vi "AlliGator Fit Method Benchmark.vi"() -> ()   [LabVIEW 2021, in "AlliGator Fit Method Benchmark.lvlib"]
doc: "Fit Method Benchmark GUI."
uses:
  AlliGator Fit Method Benchmark.lvlib
  AlliGator Fit Simulation Parameters.ctl
  AlliGator Decay Simulation Parameters.ctl
  Arrays/Array Statistics.ctl
  Fits/Decay Convolution/Decay Model.ctl
  Fits/Residual Type.ctl
  Fits/IRF(X)PSED/Fit Weights Type.ctl
  Fits/Non-linear Fitting Method v2.ctl
  Fits/Fit Calculation Method.ctl
  Fits/Non-linear Fitting Algorithm.ctl
  AlliGator Decay Fit Parameter Constraints 2.ctl
  Fits/IRF(X)PSED/Decay Fit Parameters In List.ctl
  Fits/IRF(X)PSED/MLE Baseline Offset Type.ctl
  Fits/IRF(X)PSED/IRF(X)PSED Fit Results.ctl
  AlliGator Decay Fit Options & Parameters v2.ctl
  Fits/IRF(X)PSED/Decay Fit Options v2.ctl
  Graphs/XY Graph/XY Graph Event.ctl
  <vilib>/Utility/miscctls.llb/LVPoint32TypeDef.ctl
  1e2fc33e-f2e1-4865-bd35-b782600da79c.vi
  ffbda573-fdee-4728-9e4a-091745fb94a5.vi
  20485d49-49ee-422f-9a66-761cdf75a503.vi
  AlliGator Abort.vi
  Graphs/XY Graph/XY Graph Add Single Plot with Name.vi
  GUI/GUI.lvlib
  Notebook/Notebook.lvlib
  Error/Error.lvlib
  AlliGator Globals, Variables & Constants.lvlib
  Graphs/XY Graph/XY Graph Add-Ons.lvlib
  Fits/Fits.lvlib
  AlliGator Decay Fit.lvlib
  AlliGator Decay Fit Parameter Map.lvlib
  Utilities/Utilities.lvlib
  <vilib>/vision/NI_Vision_Development_Module.lvlib
  Arrays/Arrays.lvlib
panel:
  in  "Tab Control":T1(tab)
  in  "Export Results":bool
  in  "Histogram Lower Percentile":dbl
  in  "Histogram Upper Percentile":dbl=100.0
  out "Histograms":cluster{"Axis":dbl[], "Histogram":dbl[]}[](graph)
  in  "Run Simulation":bool
  in  "Fit Simulation Parameters":T2={"# Counts"=100, "# Simulations (N)"=100, "Decay Bin Size"=1.0000000000000002e-10, "# Bins"=200}
  in  "Decay Simulation Parameters":T3={"tau 1"=1e-09, "tau 2"=0.0, "a1"=1.0, "Baseline"=0.0}
  out "tau 1":T4 {"Min" format="%#_4g"; "Max" format="%#_4g"; "Mean" format="%#_4g"; "Standard Deviation" format="%#_4g"}
  out "tau 2":T4 {"Min" format="%#_4g"; "Max" format="%#_4g"; "Mean" format="%#_4g"; "Standard Deviation" format="%#_4g"}
  out "a1":T4 {"Min" format="%#_4g"; "Max" format="%#_4g"; "Mean" format="%#_4g"; "Standard Deviation" format="%#_4g"}
  out "Message":string caption="Output (see Notebook)"
  in  "Histogram Bin Size (a1)":dbl=0.1
  in  "Histogram Bin Size (Lifetime)":dbl[unit]=1.0000000000000002e-10
  out "# Photons":dbl[](array[numeric])
  in  "Select Decay, Fit & Residuals Index":i32=1 min=1
  out "Decay Graph":cluster{"Axis":dbl[], "Histogram":dbl[]}[](graph)
  in  "Show Decays, Fits & Residuals":bool
  out "Experimental IRF Loaded":bool
  in  "Use Experimental IRF":bool
  in  "# Logical Processors Used":i32=4 caption="Used" min=1 max=16
  out "# Logical Processors":i32
  in  "MLE Baseline Offset Type":T5
  in  "MLE Baseline Offset":dbl
  in  "Fit Parameter Constraints":T6[](array[typedef]) {"Max Value" format="%#.3g"; "Min Value" format="%#.3g"}
  in  "Decay Fit Options":T14={"Show Fit Residuals"=TRUE, "Fit Model"=enum."1-Exponential", "Residual Type"=enum."Standard", "Max Decay Percentile"=100.0, "Min Decay Percentile"=0.0, "Show Full Decay"=TRUE, "Weights"=enum."1/Variance", "Fitting Method"=enum."Least Square", "Compute Parameter Uncertainties"=TRUE, "Periodic Boundaries"=TRUE, "Model Calculation"=enum."Simulation", "Period"=1.2500000000000001e-08, "Termination Criteria"={"Max Iterations"=1000, "Max Function Calls"=10000, "Max Time"=100.0, "Function Tolerance"=1e-06, "Parameter Tolerance"=1e-06, "Gradient Tolerance"=1e-06, "Min Lambda"=1e-06, "Max Lambda"=1000000.0, "Initial Tick Count"=0}, "Offset Resolution"=5.000000000000001e-11, "Use Local IRF"=FALSE, "Fitting Algorithm"=enum."Levenberg-Marquardt"} {"Offset Resolution" min=0.0; "Period" min=0.0; "Min Decay Percentile" min=0.0 max=1.0; "Max Decay Percentile" min=0.0 max=100.0}
  in  "Animated Busy Icon":bool=TRUE
  in  "Abort":bool
  out "Progress Bar":dbl(slide) scale=0.0..100.0
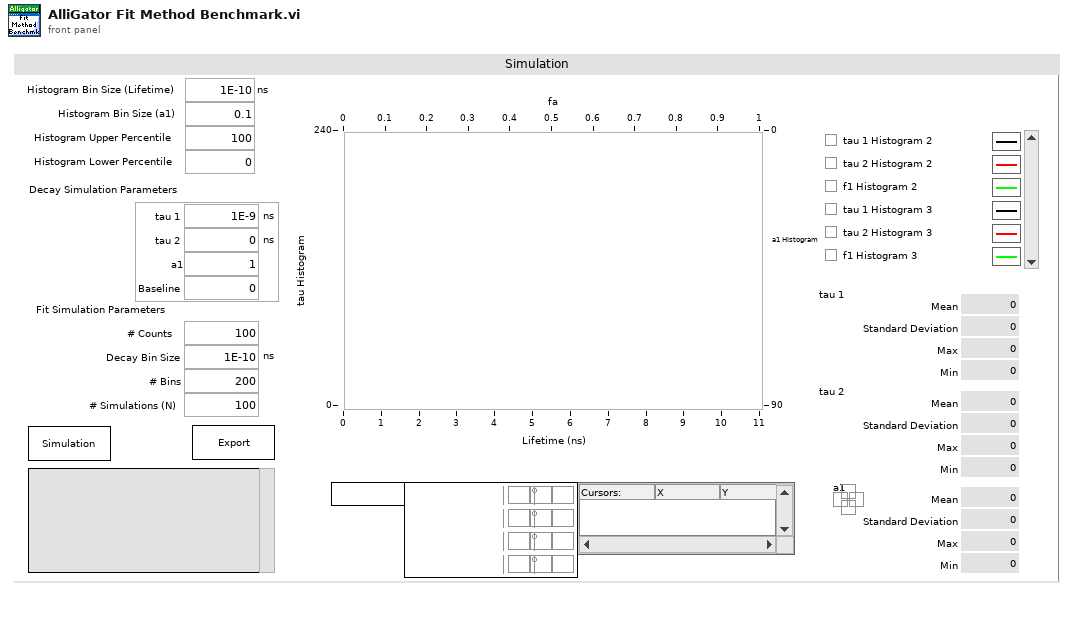
[diagram p1: front panel]
types:
  T1 = enum32{"Simulation", "Decay, Fit & Residuals Plots", "Settings"}
  T2 = typedef "AlliGator Fit Method Benchmark.lvlib/AlliGator Fit Simulation Parameters.ctl" = cluster{"# Counts":i32, "# Simulations (N)":i32, "Decay Bin Size":dbl[unit], "# Bins":i32}
  T3 = typedef "AlliGator Fit Method Benchmark.lvlib/AlliGator Decay Simulation Parameters.ctl" = cluster{"tau 1":dbl[unit], "tau 2":dbl[unit], "a1":dbl, "Baseline":dbl}
  T4 = typedef "Arrays.lvlib/Array Statistics.ctl" = cluster{"Mean":dbl, "Standard Deviation":dbl, "Max":dbl, "Min":dbl}
  T5 = typedef "Fits.lvlib/MLE Baseline Offset Type.ctl" = enum32{"Absolute", "Percentage"}
  T6 = typedef "AlliGator Decay Analysis.lvlib/AlliGator Decay Fit.lvlib/AlliGator Decay Fit Parameter Constraints 2.ctl" = cluster{"Fit Parameter":T7, "Min Value":dbl, "Max Value":dbl, "Global":bool, "Used":bool}
  T7 = typedef "Fits.lvlib/Decay Fit Parameters In List.ctl" = enum16{"Offset", "Baseline", "A_1", "tau_1", "A_2", "tau_2"}
  T8 = typedef "Fits.lvlib/Decay Model.ctl" = enum16{"1-Exponential", "2-Exponentials"}
  T9 = typedef "Fits.lvlib/Residual Type.ctl" = enum16{"Standard", "Normalized", "Reduced"}
  T10 = typedef "Fits.lvlib/Fit Weights Type.ctl" = enum16{"Unweighted", "1/Variance", "Best of All"}
  T11 = typedef "Fits.lvlib/Non-linear Fitting Method v2.ctl" = enum16{"Least Square", "Least Absolute Residual", "Bisquare", "MLE", "-", "Best of All"}
  T12 = typedef "Fits.lvlib/Fit Calculation Method.ctl" = enum16{"Simulation", "Convolution", "Integration"}
  T13 = typedef "Fits.lvlib/Non-linear Fitting Algorithm.ctl" = enum16{"Levenberg-Marquardt", "Trust-Region Dogleg"}
  T14 = cluster{"Show Fit Residuals":bool, "Fit Model":T8, "Residual Type":T9, "Max Decay Percentile":dbl, "Min Decay Percentile":dbl, "Show Full Decay":bool, "Weights":T10, "Fitting Method":T11, "Compute Parameter Uncertainties":bool, "Periodic Boundaries":bool, "Model Calculation":T12, "Period":dbl[unit], "Termination Criteria":cluster{"Max Iterations":i32, "Max Function Calls":i32, "Max Time":dbl[unit], "Function Tolerance":dbl, "Parameter Tolerance":dbl, "Gradient Tolerance":dbl, "Min Lambda":dbl, "Max Lambda":dbl, "Initial Tick Count":u32}, "Offset Resolution":dbl[unit], "Use Local IRF":bool, "Fitting Algorithm":T13}
  T15 = typedef "XY Graph Add-Ons.lvlib/XY Graph Refnum.ctl" = refnum<vi>
  T16 = typedef "AlliGator Progress Bar Q Element.ctl" = cluster{"Action":string, "Value":dbl}
  T17 = typedef "Fits.lvlib/IRF(X)PSED Fit Results.ctl" = cluster{"Best Fit Parameters (All)":dbl[], "Delta Best Fit Parameters (All)":dbl[], "R^2":dbl, "Reduced Chi^2":dbl}
  T18 = typedef "AlliGator Decay Fit Parameter Map.lvlib/AlliGator Decay Fit Options & Parameters v2.ctl" = cluster{"SYNC Period":dbl[unit], "Fit Options":T19, "Fit Parameter Constraints":T6[], "MLE Baseline Offset":dbl, "MLE Baseline Offset Type":T5}
  T19 = typedef "Fits.lvlib/Decay Fit Options v2.ctl" = cluster{"Show Fit Residuals":bool, "Fit Model":T8, "Residual Type":T9, "Max Decay Percentile":dbl, "Min Decay Percentile":dbl, "Show Full Decay":bool, "Weights":T10, "Fitting Method":T11, "Compute Parameter Uncertainties":bool, "Periodic Boundaries":bool, "Model Calculation":T12, "Period":dbl[unit], "Termination Criteria":cluster{"Max Iterations":i32, "Max Function Calls":i32, "Max Time":dbl[unit], "Function Tolerance":dbl, "Parameter Tolerance":dbl, "Gradient Tolerance":dbl, "Min Lambda":dbl, "Max Lambda":dbl, "Initial Tick Count":u32}, "Offset Resolution":dbl[unit], "Use Local IRF":bool, "Fitting Algorithm":T13}
  T20 = typedef "XY Graph Add-Ons.lvlib/XY Graph Event.ctl" = cluster{"Item Tag":string, "XY Graph Refnum":refnum<vi>, "Coords":T21, "Item Path":string}
  T21 = typedef "LVPoint32TypeDef.ctl" = cluster{"Horizontal":i32, "Vertical":i32}
  T22 = typedef "XY Graph Add-Ons.lvlib/XY Plot Data.ctl" = cluster{"X Array":dbl[], "Y Array":dbl[]}
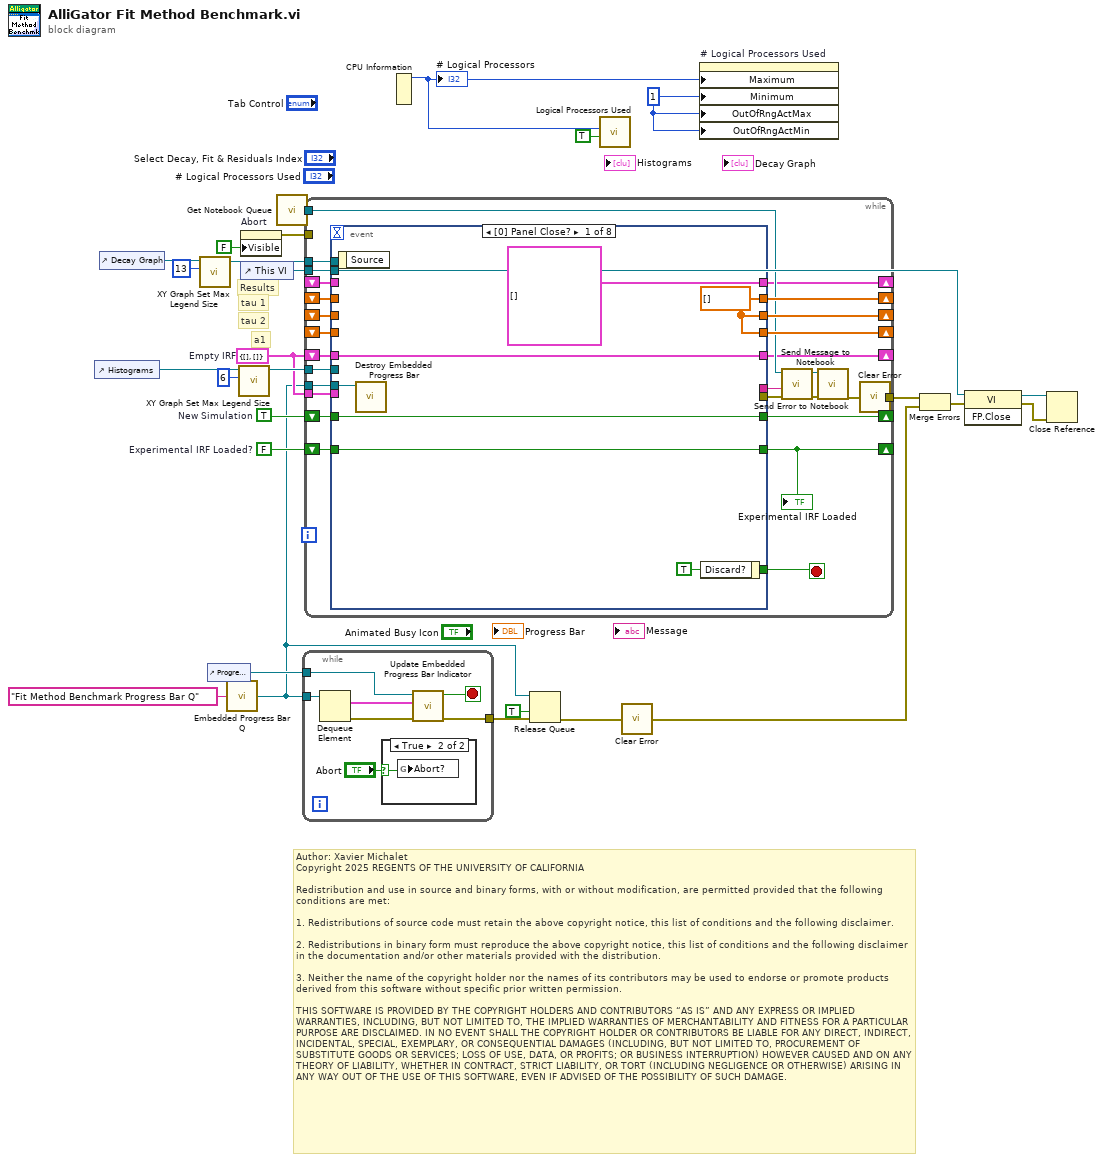
[diagram p0: block diagram]
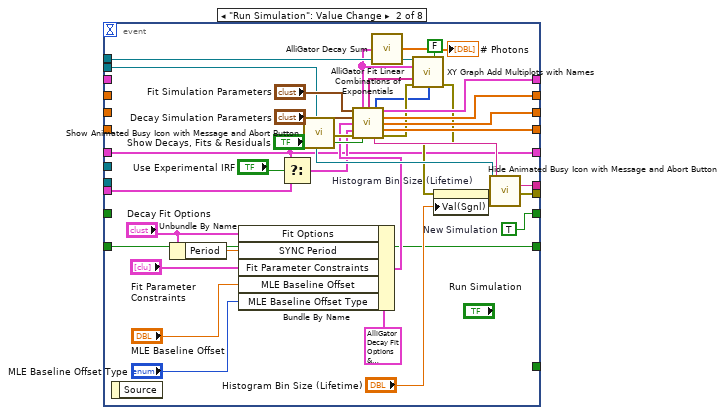
[diagram p3: hidden frame]
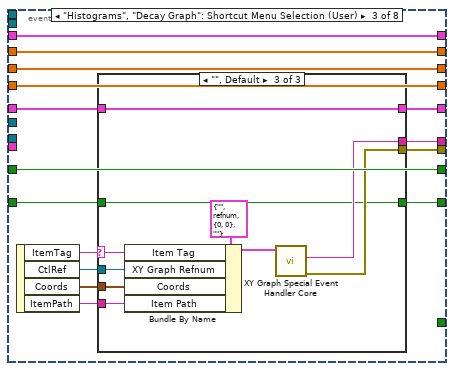
[diagram p4: hidden frame]
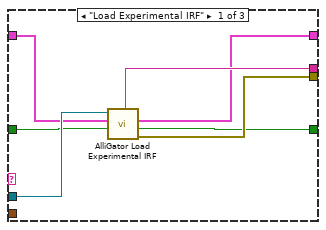
[diagram p5: hidden frame]
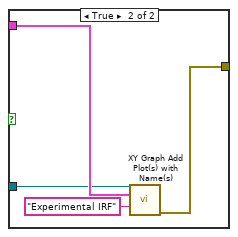
[diagram p7: hidden frame]
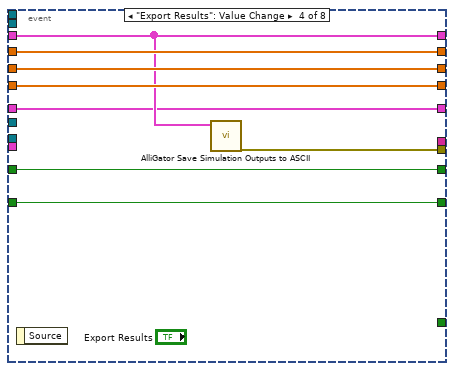
[diagram p8: hidden frame]
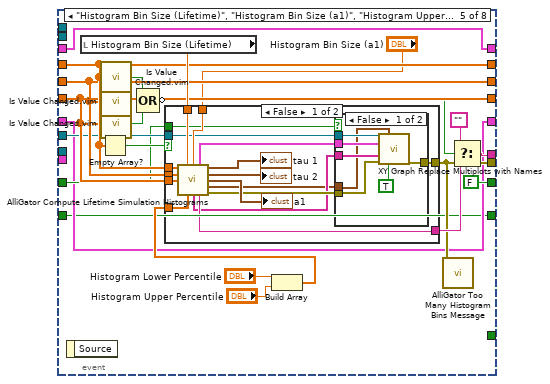
[diagram p9: hidden frame]
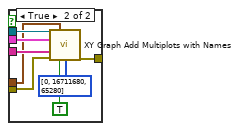
[diagram p10: hidden frame]
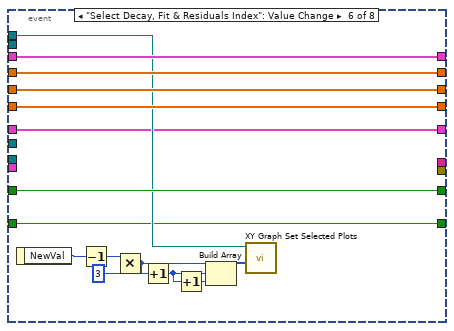
[diagram p12: hidden frame]
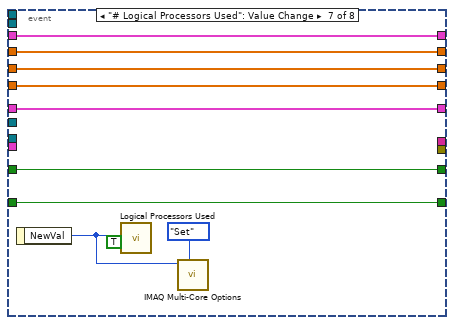
[diagram p13: hidden frame]
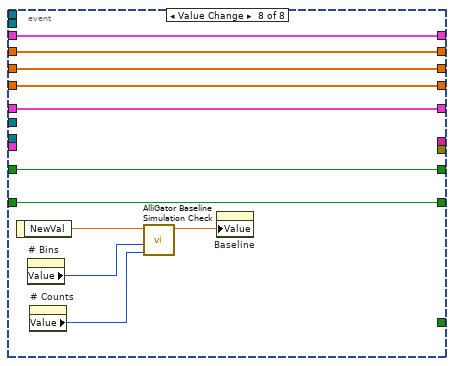
[diagram p14: hidden frame]
diagram:
  w3 = FALSE  # Experimental IRF Loaded?
  w4 = cluster{"t Array":dbl[], "IRF Array":dbl[]} {"t Array"=[], "IRF Array"=[]}  # Empty IRF
  w5 = u8 1 ("Data Entry Limits:Minimum")
  w8 = TRUE  # New Simulation
  # "Author: Xavier Michalet\nCopyright 2025 REGENTS OF THE UNIVERSITY OF CALIFORNIA\n\nRedistribution and use in source and binary forms, with or without modification, are permitted provided that the following conditions are met:\n\n1. Redistributions of source code must retain the above copyright notice, this list of conditions and the following disclaimer.\n\n2. Redistributions in binary form must reproduce the above copyright notice, this list of conditions and the following disclaimer in the documentation and/or other materials provided with the distribution.\n\n3. Neither the name of the copyright holder nor the names of its contributors may be used to endorse or promote products derived from this software without specific prior written permission.\n\nTHIS SOFTWARE IS PROVIDED BY THE COPYRIGHT HOLDERS AND CONTRIBUTORS “AS IS” AND ANY EXPRESS OR IMPLIED WARRANTIES, INCLUDING, BUT NOT LIMITED TO, THE IMPLIED WARRANTIES OF MERCHANTABILITY AND FITNESS FOR A PARTICULAR PURPOSE ARE DISCLAIMED. IN NO EVENT SHALL THE COPYRIGHT HOLDER OR CONTRIBUTORS BE LIABLE FOR ANY DIRECT, INDIRECT, INCIDENTAL, SPECIAL, EXEMPLARY, OR CONSEQUENTIAL DAMAGES (INCLUDING, BUT NOT LIMITED TO, PROCUREMENT OF SUBSTITUTE GOODS OR SERVICES; LOSS OF USE, DATA, OR PROFITS; OR BUSINESS INTERRUPTION) HOWEVER CAUSED AND ON ANY THEORY OF LIABILITY, WHETHER IN CONTRACT, STRICT LIABILITY, OR TORT (INCLUDING NEGLIGENCE OR OTHERWISE) ARISING IN ANY WAY OUT OF THE USE OF THIS SOFTWARE, EVEN IF ADVISED OF THE POSSIBILITY OF SUCH DAMAGE."
  # "Results"
  # "a1"
  # "tau 2"
  # "tau 1"
  n1 = control-ref of="Histograms"() -> (w14:refnum<vi>)
  n2 = control-ref of="Decay Graph"() -> (w11:refnum<vi>)
  n3 = call "XY Graph Set Max Legend Size.vi"("Max Legend Size"=13, "XY Graph Refnum"=w11) -> ("XY Graph Refnum (dup)"=w10:T15)  [unwired: 8 in, 1 out]
  n4 = control-ref of="Progress Bar"() -> (w26:refnum<vi>)
  n5 = call "Embedded Progress Bar Q.vi"("Progress Bar Queue Name"="Fit Method Benchmark Progress Bar Q") -> ("Progress Bar Queue"=w1:refnum<queue>)  [unwired: 6 in]
  n6 = call "XY Graph Set Max Legend Size.vi"("Max Legend Size"=6, "XY Graph Refnum"=w14) -> ("XY Graph Refnum (dup)"=w12:T15)  [unwired: 8 in, 1 out]
  n7 = property on="Abort" class="Bool"("Visible"=FALSE) -> (error out=w16:errorcluster)  [unwired: 2 in, 1 out]
  n8 = control-ref of="This VI"() -> (w15:refnum<vi>)
  n9 = call "Get Notebook Queue.vi"() -> ("Notebook Queue"=w23:refnum<queue>)  [unwired: 9 in]
  n10 = while {
    tunnel: w1 -> [w34]
    tunnel: w26 -> [w32]
    tunnel: [w29] -> w25
    stop <- w30 stop-if-true
    n11 = Dequeue Element(queue=w34) -> (element=w33:T16, error out=w31:errorcluster)  [unwired: 2 in, 2 out]
    n12 = case shown="True" "Abort" {
      selector: "Abort" -> [_ w35]
      frame False {
      }
      frame True {
        n13 = global write "AlliGator Abort.vi" "Abort?"(w35) -> ()
      }
    }
    n14 = call "Update Embedded Progress Bar Indicator.vi"("Error In"=w31, "Progress Bar Event"=w33, "Progress Bar Refnum"=w32) -> ("Error Out"=w29:errorcluster, "Quit?"=w30:bool)  [unwired: 7 in]
  }
  n15 = while {
    shift-right: [w61] -> _
    shift-left: _ -> [w58]
    shift-right: [w60] -> _
    shift-left: _ -> [w57]
    shift-right: [w59] -> _
    shift-left: _ -> [w56]
    tunnel: w1 -> [w55]
    tunnel: w23 -> [w54]
    tunnel: [w48] -> w22
    tunnel: w16 -> [_]
    tunnel: w15 -> [w47]
    tunnel: w12 -> [w46]
    shift-right: [w45] -> _
    shift-left: _ -> [w44]
    tunnel: w10 -> [w43]
    shift-right: [w41] -> _
    shift-left: w8 -> [w42]
    shift-right: [w39] -> _
    shift-left: w4 -> [w40]
    tunnel: w4 -> [w38]
    shift-right: [w36] -> _
    shift-left: w3 -> [w37]
    stop <- w62 stop-if-true
    n16 = event shown="[0] Panel Close?" {
      selector: _ -> [_ _ _ _ _ _ _ _]
      dyn-events: _ -> [_ _ _ _ _ _ _ _]
      timeout: _ -> [_ _ _ _ _ _ _ _]
      tunnel: [w69 _ _ _ _ _ _ _] -> w62
      tunnel: [w66 w101 w118 w151 w172 w221 w231 w242] -> w61
      tunnel: [w66 w100 w117 w150 w171 w220 w230 w241] -> w60
      tunnel: [w66 w99 w116 w149 w170 w219 w229 w240] -> w59
      tunnel: w58 -> [_ _ w118 w151 w172 w221 w231 w242]
      tunnel: w57 -> [_ _ w117 w150 w171 w220 w230 w241]
      tunnel: w56 -> [_ _ w116 w149 w170 w219 w229 w240]
      tunnel: w55 -> [w68 _ _ _ _ _ _ _]
      tunnel: [_ w94 w111 _ w164 _ _ _] -> w53
      tunnel: [_ w95 w110 w146 w154 _ _ _] -> w49
      tunnel: w47 -> [_ w82 _ _ _ _ _ _]
      tunnel: w46 -> [_ _ _ _ w159 _ _ _]
      tunnel: [T17[] [] ("Fit Results") w89 w109 w147 w158 w218 w228 w239] -> w45
      tunnel: w44 -> [_ _ w109 w147 w158 w218 w228 w239]
      tunnel: w43 -> [_ w86 _ _ _ w216 _ _]
      tunnel: w42 -> [w65 _ w108 w148 w156 w217 w227 w238]
      tunnel: [w65 w78 w108 w148 FALSE ("New Simulation") w217 w227 w238] -> w41
      tunnel: w40 -> [w64 w74 w107 w145 w153 w208 w223 w233]
      tunnel: [w64 w74 w106 w145 w153 w208 w223 w233] -> w39
      tunnel: w38 -> [_ w73 _ _ _ _ _ _]
      tunnel: w37 -> [w63 w72 w105 w144 w152 w207 w222 w232]
      tunnel: [w63 w72 w104 w144 w152 w207 w222 w232] -> w36
      event Panel Close? {
        w66 = dbl[] [] ("tau 1")
        w69 = TRUE ("Discard?")
        n17 = event-data() -> ()  [unwired: 1 in, 1 out]
        n18 = call "Destroy Embedded Progress Bar.vi"("Progress Bar Queue in"=w68) -> ()  [unwired: 10 in, 1 out]
        n19 = event-data("Discard?"=w69) -> ()  [unwired: 1 in, 1 out]
      }
      event "Run Simulation": Value Change {
        w78 = TRUE  # New Simulation
        n20 = event-data() -> ()  [unwired: 1 in, 1 out]
        n21 = Unbundle By Name("Decay Fit Options") -> ("Period"=w93:dbl[unit])
        n22 = Bundle By Name(cluster=T18 {"SYNC Period"=0.0, "Fit Options"={"Show Fit Residuals"=FALSE, "Fit Model"=enum."1-Exponential", "Residual Type"=enum."Standard", "Max Decay Percentile"=0.0, "Min Decay Percentile"=0.0, "Show Full Decay"=FALSE, "Weights"=enum."Unweighted", "Fitting Method"=enum."Least Square", "Compute Parameter Uncertainties"=FALSE, "Periodic Boundaries"=FALSE, "Model Calculation"=enum."Simulation", "Period"=0.0, "Termination Criteria"={"Max Iterations"=0, "Max Function Calls"=0, "Max Time"=0.0, "Function Tolerance"=0.0, "Parameter Tolerance"=0.0, "Gradient Tolerance"=0.0, "Min Lambda"=0.0, "Max Lambda"=0.0, "Initial Tick Count"=0}, "Offset Resolution"=0.0, "Use Local IRF"=FALSE, "Fitting Algorithm"=enum."Levenberg-Marquardt"}, "Fit Parameter Constraints"=[], "MLE Baseline Offset"=0.0, "MLE Baseline Offset Type"=enum."Absolute"} ("Decay Fit Options & Parameters"), "Fit Options"="Decay Fit Options", "SYNC Period"=w93, "Fit Parameter Constraints"="Fit Parameter Constraints", "MLE Baseline Offset"="MLE Baseline Offset", "MLE Baseline Offset Type"="MLE Baseline Offset Type") -> (w81:T18)
        n23 = Select(t=w74, s="Use Experimental IRF", f=w73) -> (s? t:f=w75:T22)
        n24 = call "Show Animated Busy Icon with Message and Abort Button.vi"("Target VI reference"=w82) -> ("Error Out"=w97:errorcluster)  [unwired: 18 in]
        n25 = call "AlliGator Fit Linear Combinations of Exponentials.vi"("Fit Simulation Parameters"="Fit Simulation Parameters", "Decay Simulation Parameters"="Decay Simulation Parameters", "Decay Fit Options & Parameters"=w81, "Reference Decay"=w75, "Error In"=w97, "Show Decays, Fits & Residuals"="Show Decays, Fits & Residuals") -> ("Output Plots"=w71:cluster{"t Array":dbl[], "I Array":dbl[]}[], "Output Plot Names"=w85:string[], "Plot Colors"=w84:u32[], "Fit Results"=w89:T17[], "tau 1"=w101:dbl[], "tau 2"=w100:dbl[], "a 1"=w99:dbl[], "Message"=w94:string, "Error Out"=w87:errorcluster)  [unwired: 1 in]
        n26 = call "AlliGator Decay Sum.vi"("Output Plots"=w71) -> ("# Photons"=→"# Photons":dbl[])
        n27 = call "XY Graph Add Multiplots with Names.vi"("XYGraph in"=w86, "Keep Existing Plots (T)"=FALSE, "Array of Plots"=w71, "Array of Plot Names (\"Plot\")"=w85, "error in (no error)"=w87, "Plot Colors (Default)"=w84) -> ("error out"=w77:errorcluster)  [unwired: 5 in, 4 out]
        n28 = property on="Histogram Bin Size (Lifetime)" class="DigNum (strict)"(error in=w77, "Val(Sgnl)"="Histogram Bin Size (Lifetime)") -> (error out=w96:errorcluster)  [unwired: 1 in, 1 out]
        n29 = call "Hide Animated Busy Icon with Message and Abort Button.vi"("Message"=w94, "Target VI reference"=w82, "Error In"=w96) -> ("Error Out"=w95:errorcluster)  [unwired: 16 in]
      }
      event "Histograms", "Decay Graph": Shortcut Menu Selection (User) {
        n30 = event-data() -> ("ItemTag"=w115:string, "CtlRef"=w114:refnum<vi>, "Coords"=w113:T21, "ItemPath"=w112:string)  [unwired: 1 in]
        n31 = case shown="\"\", Default" w115 {
          selector: w115 -> [_ _ w142]
          tunnel: w114 -> [w125 w127 w141]
          tunnel: w113 -> [_ _ w140]
          tunnel: w112 -> [_ _ w139]
          tunnel: [w123 _ w137] -> w111
          tunnel: [w124 w126 w136] -> w110
          tunnel: w107 -> [w120 w128 w135]
          tunnel: [w119 w128 w135] -> w106
          tunnel: w105 -> [w121 w129 w134]
          tunnel: [w122 w129 w134] -> w104
          frame "Load Experimental IRF" {
            n32 = call "AlliGator Load Experimental IRF.vi"("Experimental IRF Loaded?"=w121, "Plot Data in"=w120, "XYGraph in"=w125) -> ("error out"=w124:errorcluster, "Experimental IRF Loaded?"=w122:bool, "Plot Data out"=w119:T22, "Message"=w123:string)  [unwired: 5 in]
          }
          frame "Show Experimental IRF" {
            n33 = case shown="False" w129 {
              tunnel: w128 -> [_ w133]
              tunnel: w127 -> [_ w132]
              tunnel: [_ w130] -> w126
              frame False {
              }
              frame True {
                n34 = call-poly "XY Graph Add Plot(s) with Name(s).vi"("XYGraph Ref in"=w132, "Plot"=w133, "Plot Name (\"Plot\")"="Experimental IRF" ("Plot Name (\"Plot\")")) -> ("error out"=w130:errorcluster)  [unwired: 9 in, 3 out]
              }
            }
          }
          frame "", Default {
            n35 = Bundle By Name(cluster=T20 {"Item Tag"="", "XY Graph Refnum"=refnum, "Coords"={"Horizontal"=0, "Vertical"=0}, "Item Path"=""} ("XY Graph Event"), "Item Tag"=w142, "XY Graph Refnum"=w141, "Coords"=w140, "Item Path"=w139) -> (w138:T20)
            n36 = call "XY Graph Special Event Handler Core.vi"("XY Graph Event"=w138) -> ("error out"=w136:errorcluster, "Message"=w137:string)  [unwired: 6 in, 3 out]
          }
        }
      }
      event "Export Results": Value Change {
        n37 = event-data() -> ()  [unwired: 1 in, 1 out]
        n38 = call "AlliGator Save Simulation Outputs to ASCII.vi"("Fit Results"=w147) -> ("Error Out"=w146:errorcluster)  [unwired: 10 in]
      }
      event "Histogram Bin Size (Lifetime)", "Histogram Bin Size (a1)", "Histogram Upper Percentile", "Histogram Lower Percentile": Value Change {
        n39 = event-data() -> ()  [unwired: 1 in, 1 out]
        n40 = local read "Histogram Bin Size (Lifetime)"() -> (w174:dbl[unit])
        n41 = Empty Array?(array=w172) -> (empty?=w173:bool)
        n42 = call "Is Value Changed.vim"("value"=w172) -> ("changed or first call?"=w169:bool)
        n43 = call "Is Value Changed.vim"("value"=w171) -> ("changed or first call?"=w168:bool)
        n44 = call "Is Value Changed.vim"("value"=w170) -> ("changed or first call?"=w167:bool)
        n45 = Compound Arithmetic op=OR(w169, w168, w167) -> (invert w166:bool)
        n46 = Build Array("Histogram Lower Percentile", "Histogram Upper Percentile") -> (w160:dbl[])
        n47 = case shown="False" w173 {
          tunnel: w174 -> [w191 _]
          tunnel: w171 -> [w190 _]
          tunnel: w170 -> [w189 _]
          tunnel: w172 -> [w188 _]
          tunnel: [w184 _] -> w165
          tunnel: [w178 _] -> w154
          tunnel: "Histogram Bin Size (a1)" -> [w183 _]
          tunnel: w160 -> [w182 _]
          tunnel: w159 -> [w181 _]
          tunnel: w156 -> [w176 _]
          frame False {
            n48 = call "AlliGator Compute Lifetime Simulation Histograms.vi"("tau 1"=w188, "Histogram Bin Size (tau)"=w191, "Histogram Bin Size (f1)"=w183, "tau 2"=w190, "a1"=w189, "Percentiles to Keep (1, 99)"=w182) -> ("Histograms"=w180:cluster{"Axis":dbl[], "Histogram":dbl[]}[], "Array Statistic (tau 1)"=→"tau 1":T4, "Array Statistics (tau 2)"=→"tau 2":T4, "Array Statistics (a1)"=→"a1":T4, "Array of Scales"=w175:cluster{"X Scale":u32, "Y Scale":u32}[], "Plot Names"=w177:string[], "Message"=w184:string, "Error Out"=w179:errorcluster)  [unwired: 2 in]
            n49 = case shown="False" w176 {
              tunnel: w181 -> [w198 w206]
              tunnel: w180 -> [w197 w205]
              tunnel: w179 -> [w195 w204]
              tunnel: [w194 w203] -> w178
              tunnel: w177 -> [w196 w201]
              tunnel: w175 -> [w192 w200]
              frame False {
                n50 = call "XY Graph Replace Multiplots with Names.vi"("XYGraph in"=w198, "Array of Scales (Default)"=w192, "Array of Plots"=w197, "Array of Plot Names (\"Plot\")"=w196, "error in (no error)"=w195, "Make Visible (T)"=TRUE) -> ("error out"=w194:errorcluster)  [unwired: 5 in, 4 out]
              }
              frame True {
                n51 = call "XY Graph Add Multiplots with Names.vi"("XYGraph in"=w206, "Array of Scales (Default)"=w200, "Array of Plots"=w205, "Array of Plot Names (\"Plot\")"=w201, "error in (no error)"=w204, "Make Visible (T)"=TRUE, "Plot Colors (Default)"=u32[] [0, 16711680, 65280]) -> ("error out"=w203:errorcluster)  [unwired: 4 in, 4 out]
              }
            }
          }
          frame True {
          }
        }
        n52 = call "AlliGator Too Many Histogram Bins Message.vi"("error in (no error)"=w154) -> ()
        n53 = Select(t="", s=w166, f=w165) -> (s? t:f=w164:string)
      }
      event "Select Decay, Fit & Residuals Index": Value Change {
        n54 = event-data() -> ("NewVal"=w215:i32)  [unwired: 1 in]
        n55 = Decrement(x=w215) -> (x-1=w214:i32)
        n56 = Multiply(x=w214, y=3) -> (x*y=w211:i32)
        n57 = Increment(x=w211) -> (x+1=w210:i32)
        n58 = Increment(x=w210) -> (x+1=w209:i32)
        n59 = Build Array(w211, w210, w209) -> (w212:i32[])
        n60 = call "XY Graph Set Selected Plots.vi"("Selected Plots"=w212, "XY Graph Refnum"=w216) -> ()  [unwired: 6 in, 4 out]
      }
      event "# Logical Processors Used": Value Change {
        n61 = event-data() -> ("NewVal"=w224:i32)  [unwired: 1 in]
        n62 = call "Logical Processors Used.vi"("Set/Get (F)"=TRUE, "# Logical Processor Used"=w224) -> ()  [unwired: 4 in, 1 out]
        n63 = call "IMAQ Multi-Core Options"("Get/Set Number of Cores (Get)"=enum32{"Get", "Set", "Set Max Available"}."Set", "Specified Number of Cores"=w224) -> ()  [unwired: 8 in, 2 out]
      }
      event Value Change {
        n64 = event-data() -> ("NewVal"=w237:dbl)  [unwired: 1 in]
        n65 = property on="# Bins" class="DigNum (strict)"() -> ("Value"=w236:i32)  [unwired: 2 in, 2 out]
        n66 = property on="# Counts" class="DigNum (strict)"() -> ("Value"=w235:i32)  [unwired: 2 in, 2 out]
        n67 = call "AlliGator Baseline Simulation Check.vi"("# Counts"=w235, "# Bins"=w236, "New Baseline in"=w237) -> ("New Baseline out"=w234:dbl)  [unwired: 8 in]
        n68 = property on="Baseline" class="DigNum (strict)"("Value"=w234) -> ()  [unwired: 2 in, 2 out]
      }
    }
    "Experimental IRF Loaded" <- w36
    n69 = call "Send Message to Notebook.vi"("Error In"=w49, "Message"=w53, "Notebook Queue"=w54) -> ("Error Out"=w51:errorcluster, "Notebook Queue"=w52:refnum<queue>)  [unwired: 5 in]
    n70 = call "Send Error to Notebook.vi"("error in (no error)"=w51, "Notebook Q"=w52) -> ("Error Out"=w50:errorcluster)  [unwired: 9 in]
    n71 = call "Clear Error.vi"("Error In"=w50) -> ("no Error Out"=w48:errorcluster)  [unwired: 8 in]
  }
  n72 = CPU Information() -> (4:w7:i32)  [unwired: 3 out]
  "# Logical Processors" <- w7
  n73 = Release Queue(queue=w1, force destroy? (F)=TRUE, error in (no error)=w25) -> (error out=w21:errorcluster)  [unwired: 2 out]
  n74 = call "Logical Processors Used.vi"("Set/Get (F)"=TRUE, "# Logical Processor Used"=w7) -> ()  [unwired: 4 in, 1 out]
  n75 = call "Clear Error.vi"("Error In"=w21) -> ("no Error Out"=w2:errorcluster)  [unwired: 8 in]
  n76 = property on="# Logical Processors Used" class="DigNum (strict)"("Maximum"=w7, "Minimum"=w5, "OutOfRngActMax"=w5, "OutOfRngActMin"=w5) -> ()  [unwired: 2 in, 2 out]
  n77 = Merge Errors(w22, w2) -> (w20:errorcluster)
  n78 = invoke class="VI" method="FP.Close"(reference=w15, error in=w20) -> (reference out=w19:refnum<vi>, error out=w18:errorcluster)  [unwired: 1 in, 1 out]
  n79 = Close Reference(reference=w19, error in (no error)=w18) -> ()  [unwired: 1 out]
